vi "pmu_Get Reporting Time Information.vi"(0 "timestamps in":dbl[][](array[numeric]), 1 "reset? (F)":bool, 5 "GPS information in":T1[](array[typedef]), 7 "performance class":enum8{"M Class", "P Class"}(ring), 9 "window length":i32, 11 "reporting rate":i16, 12 "initial samples to read":u32) -> (2 "min final timestamp":timestamp, 3 "empty?":bool, 4 "timestamps out":dbl[][](array[numeric]), 6 "GPS information out":T1[](array[typedef]), 8 "max t0 index":i32, 10 "samples to read":u32, 14 "current reporting time":timestamp format="%<%.9X\n%x>T")   [LabVIEW 2013, in "NI_EP_PMU.lvlib"]
uses:
  <vilib>/addons/Electrical Power/PMU/NI_EP_PMU.lvlib
  <vilib>/addons/Electrical Power/PMU/Common/Controls/pmu_GPS Info.ctl
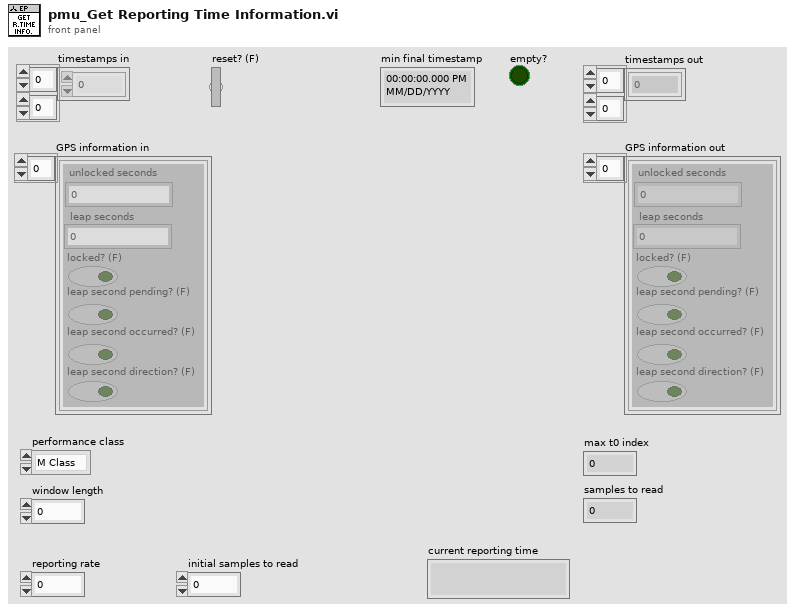
[diagram p1: front panel]
types:
  T1 = typedef "NI_EP_PMU.lvlib/pmu_GPS Info.ctl" = cluster{"unlocked seconds":u32, "leap seconds":i8, "locked? (F)":bool, "leap second pending? (F)":bool, "leap second occurred? (F)":bool, "leap second direction? (F)":bool}
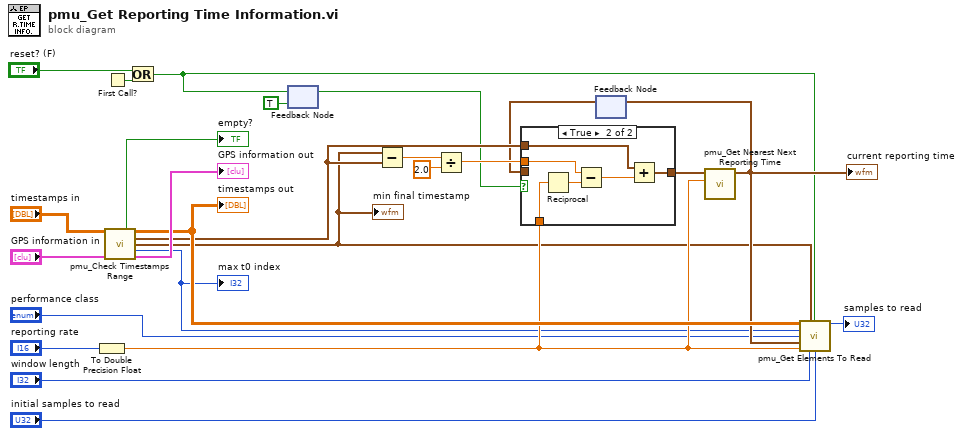
[diagram p0: block diagram]
diagram:
  n1 = To Double Precision Float(number="reporting rate") -> (double precision float=w16:dbl)
  n2 = First Call?() -> (First Call?: T/F=w6:bool)
  n3 = call <vilib>:"pmu_Check Timestamps Range.vi"("timestamps in"="timestamps in", "GPS information"="GPS information in") -> ("empty?"=→"empty?":bool, "timestamps out"=w19:dbl[][], "max initial timestamp"=w15:timestamp, "min final timestamp"=w14:timestamp, "max t0 index"=w13:i32, "buffered GPS information"=→"GPS information out":T1[])  [unwired: 8 in]
  "timestamps out" <- w19
  "max t0 index" <- w13
  "min final timestamp" <- w14
  n4 = Or(x="reset? (F)", y=w6) -> (x .or. y?=w3:bool)
  n5 = feedback #1(TRUE) -> (w2:bool)
  n6 = feedback-in #1(w3) -> ()
  n7 = Subtract(x=w14, y=w15) -> (x-y=w10:dbl)
  n8 = Divide(x=w10, y=2.0) -> (x/y=w12:dbl)
  n9 = feedback #2() -> (w11:timestamp)  [unwired: 1 in]
  n10 = case shown="True" w2 {
    tunnel: w11 -> [w26 _]
    tunnel: w15 -> [_ w30]
    tunnel: w12 -> [_ w32]
    tunnel: [w26 w29] -> w8
    tunnel: w16 -> [_ w28]
    frame False {
    }
    frame True {
      n11 = Reciprocal(x=w28) -> (1/x=w27:dbl)
      n12 = Subtract(x=w32, y=w27) -> (x-y=w31:dbl)
      n13 = Add(x=w30, y=w31) -> (x+y=w29:timestamp)
    }
  }
  n14 = call <vilib>:"pmu_Get Nearest Next Reporting Time.vi"("reporting rate"=w16, "time in"=w8) -> ("reporting time"=w18:timestamp)  [unwired: 8 in, 1 out]
  "current reporting time" <- w18
  n15 = feedback-in #2(w18) -> ()
  n16 = call <vilib>:"pmu_Get Elements To Read.vi"("timestamps"=w19, "min tfinal"=w14, "reset? (F)"=w3, "max t0 index"=w13, "performance class"="performance class", "reporting time"=w18, "reporting rate"=w16, "window length"="window length", "initial samples to read"="initial samples to read") -> ("elements to read"=→"samples to read":u32)  [unwired: 6 in]
